vi "Replot.vi"(8 "error in (no error)":errorcluster, 11 "XY WFRM Plot in":refnum<class "XY WFRM Plot.lvclass">) -> (0 "error out":errorcluster, 3 "XY WFRM Plot out":refnum<class "XY WFRM Plot.lvclass">)   [LabVIEW 2016, in "XY WFRM Plot.lvclass"]
uses:
  XY WFRM Plot.lvclass
  D:/github/Measure_core/Plots/Plot/Plot.lvclass
  Plot/Plot.lvclass/Plot.ctl
  XY WFRM Plot.lvclass/XY WFRM Plot.ctl
  Plot/Read Files.vi
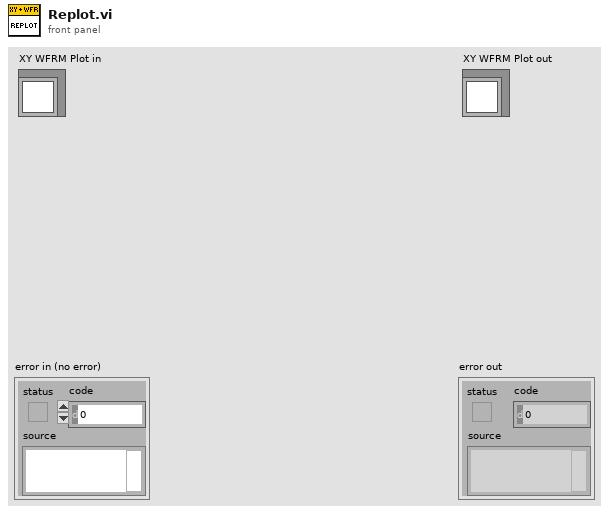
[diagram p1: front panel]
types:
  T1 = typedef "Plot types.ctl" = enum16{"Waveform Plot", "XY Plot", "Full XY"}
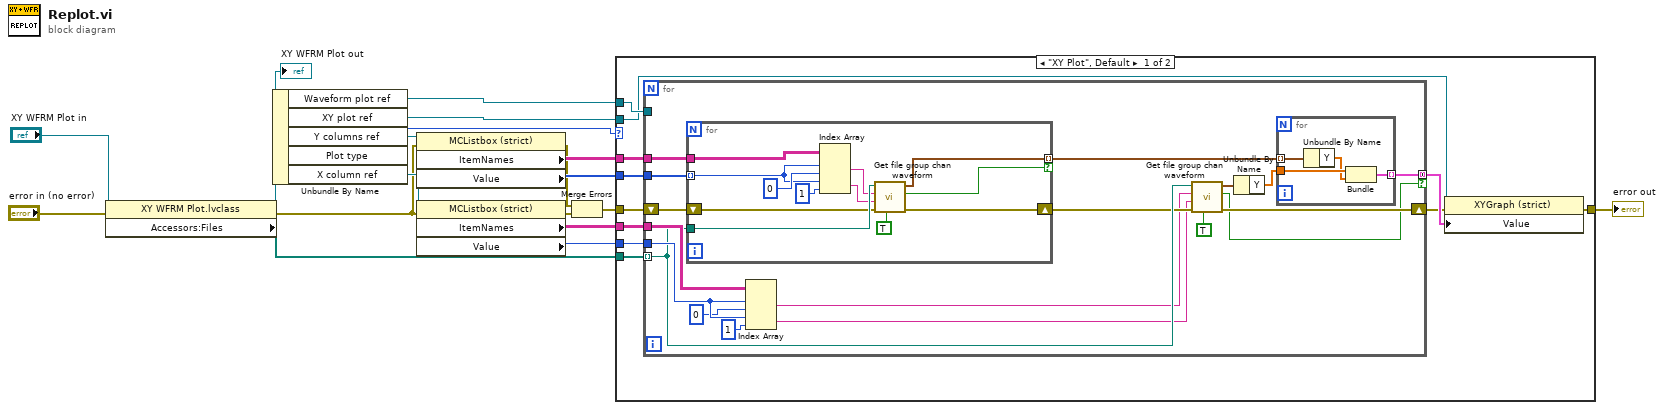
[diagram p0: block diagram]
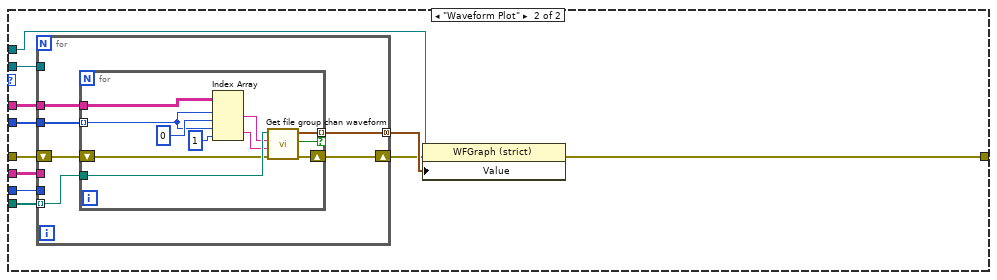
[diagram p2: hidden frame]
diagram:
  n1 = property class="XY WFRM Plot.lvclass"(reference="XY WFRM Plot in", error in="error in (no error)") -> (reference out=w5:refnum<class "XY WFRM Plot.lvclass">, error out=w7:errorcluster, "Accessors:Files"=w14:path[])
  "XY WFRM Plot out" <- w5
  n2 = Unbundle By Name(w5) -> ("Waveform plot ref"=w9:refnum<vi>, "XY plot ref"=w10:refnum<vi>, "Y columns ref"=w17:refnum<vi>, "Plot type"=w4:T1, "X column ref"=w13:refnum<vi>)
  n3 = property class="MCListbox (strict)"(reference=w17, error in=w7) -> (error out=w3:errorcluster, "ItemNames"=w16:string[][], "Value"=w15:i32[])  [unwired: 1 out]
  n4 = property class="MCListbox (strict)"(reference=w13, error in=w7) -> (error out=w2:errorcluster, "ItemNames"=w11:string[][], "Value"=w12:i32)  [unwired: 1 out]
  n5 = Merge Errors(w3, w2) -> (w1:errorcluster)
  n6 = case shown="\"XY Plot\", Default" w4 {
    tunnel: w16 -> [w29 w74]
    tunnel: w15 -> [w28 w73]
    tunnel: w14 -> [w27 w72]
    tunnel: w12 -> [w26 w71]
    tunnel: w11 -> [w25 w70]
    tunnel: w10 -> [w20 w69]
    tunnel: w9 -> [w24 w65]
    tunnel: [w21 w66] -> w6
    tunnel: w1 -> [w19 w64]
    frame "XY Plot", Default {
      n7 = for {
        tunnel: w29 -> [w47]
        tunnel: w28 -> [w46]
        tunnel: w27 -> [w42] mode=indexing
        shift-right: [w32] -> w22
        shift-left: w19 -> [w45]
        tunnel: w26 -> [w44]
        tunnel: w25 -> [w43]
        tunnel: w24 -> [_]
        tunnel: [w33] -> w23 mode=concatenating if=w31
        n8 = for {
          tunnel: w47 -> [w63]
          tunnel: w46 -> [w61] mode=indexing
          tunnel: w42 -> [w59]
          shift-right: [w54] -> w40
          shift-left: w45 -> [w56]
          tunnel: [w55] -> w41 mode=indexing if=w53
          n9 = Index Array(array=w63, index (row) #1=w61, index (col) #1=0 ("disabled index (col)"), index (row) #2=w61, index (col) #2=1 ("disabled index (col)")) -> (element #1=w58:string, element #2=w57:string)
          n10 = call "Get file group chan waveform.vi"("Clear missing ch err"=TRUE, "Error In"=w56, "Channel"=w57, "Group"=w58, "File"=w59) -> ("Error Out"=w54:errorcluster, "Valid WFRM"=w53:bool, "Waveform"=w55:waveform(sgl))  [unwired: 4 in]
        }
        n11 = Index Array(array=w43, index (row) #1=w44, index (col) #1=0 ("index (col)"), index (row) #2=w44, index (col) #2=1 ("index (col)")) -> (element #1=w37:string, element #2=w36:string)
        n12 = call "Get file group chan waveform.vi"("Clear missing ch err"=TRUE, "Error In"=w40, "Channel"=w36, "Group"=w37, "File"=w42) -> ("Error Out"=w32:errorcluster, "Valid WFRM"=w31:bool, "Waveform"=w35:waveform(sgl))  [unwired: 4 in]
        n13 = Unbundle By Name(w35) -> ("Y"=w34:sgl[])
        n14 = for {
          tunnel: w34 -> [w51]
          tunnel: w41 -> [w50] mode=indexing
          tunnel: [w48] -> w33 mode=indexing
          n15 = Unbundle By Name(w50) -> ("Y"=w49:sgl[])
          n16 = Bundle("Y"=w51, "Y"=w49) -> (w48:cluster{"Y":sgl[], "Y":sgl[]})  [unwired: 1 in]
        }
      }
      n17 = property class="XYGraph (strict)"(reference=w20, error in=w22, "Value"=w23) -> (error out=w21:errorcluster)  [unwired: 1 out]
    }
    frame "Waveform Plot" {
      n18 = for {
        tunnel: w74 -> [w80]
        tunnel: w73 -> [w79]
        tunnel: w72 -> [w77] mode=indexing
        shift-right: [w76] -> w67
        shift-left: w64 -> [w78]
        tunnel: w71 -> [_]
        tunnel: w70 -> [_]
        tunnel: w69 -> [_]
        tunnel: [w75] -> w68 mode=concatenating
        n19 = for {
          tunnel: w80 -> [w91]
          tunnel: w79 -> [w89] mode=indexing
          tunnel: w77 -> [w87]
          shift-right: [w83] -> w76
          shift-left: w78 -> [w84]
          tunnel: [w82] -> w75 mode=indexing if=w81
          n20 = Index Array(array=w91, index (row) #1=w89, index (col) #1=0 ("disabled index (col)"), index (row) #2=w89, index (col) #2=1 ("disabled index (col)")) -> (element #1=w86:string, element #2=w85:string)
          n21 = call "Get file group chan waveform.vi"("Error In"=w84, "Channel"=w85, "Group"=w86, "File"=w87) -> ("Error Out"=w83:errorcluster, "Valid WFRM"=w81:bool, "Waveform"=w82:waveform(sgl))  [unwired: 5 in]
        }
      }
      n22 = property class="WFGraph (strict)"(reference=w65, error in=w67, "Value"=w68) -> (error out=w66:errorcluster)  [unwired: 1 out]
    }
  }
  "error out" <- w6
